vi "Contour Constructor.vi"(4 "Plot ID":i32, 6 "z matrix":sgl[][](array[numeric]), 8 "error in (no error)":errorcluster, 9 "y vector":sgl[][](array[numeric]), 10 "x vector":sgl[][](array[numeric]), 11 "3D Contour Datatype.lvclass in":refnum<class "3D Contour Datatype.lvclass">) -> (0 "error out":errorcluster, 3 "3D Contour Datatype.lvclass out":refnum<class "3D Contour Datatype.lvclass">)   [LabVIEW 2017, in "3D Contour Datatype.lvclass"]
uses:
  <vilib>/Math Plots/3D Math Plots/3D Contour/3D Contour Datatype/3D Contour Datatype.lvclass
  <vilib>/Math Plots/3D Math Plots/3D Contour/3D Contour Datatype/3D Contour Datatype.lvclass/3D Contour Datatype.ctl
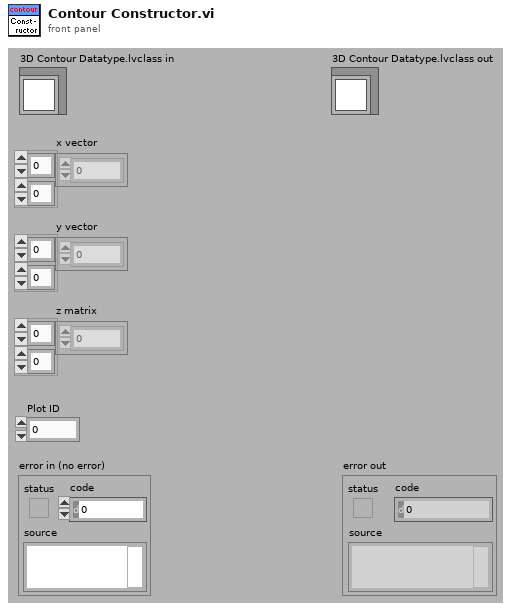
[diagram p1: front panel]
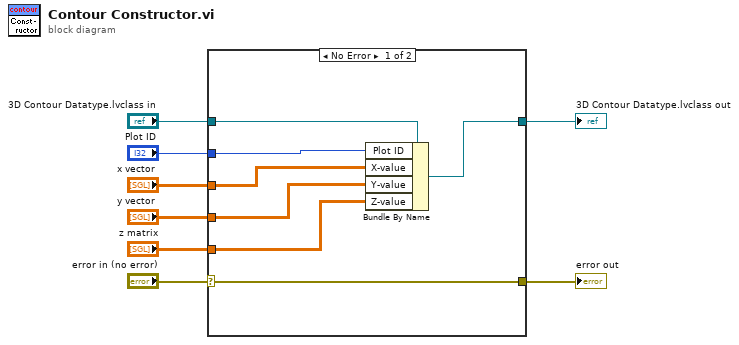
[diagram p0: block diagram]
diagram:
  n1 = case shown="No Error" "error in (no error)" {
    selector: "error in (no error)" -> [w10 w17]
    tunnel: "Plot ID" -> [w9 _]
    tunnel: [w10 w17] -> w7
    tunnel: "x vector" -> [w15 _]
    tunnel: "y vector" -> [w14 _]
    tunnel: "z matrix" -> [w13 _]
    tunnel: "3D Contour Datatype.lvclass in" -> [w12 w16]
    tunnel: [w11 w16] -> w1
    frame No Error {
      n2 = Bundle By Name(cluster=w12, "Plot ID"=w9, "X-value"=w15, "Y-value"=w14, "Z-value"=w13) -> (w11:refnum<class "3D Contour Datatype.lvclass">)
    }
    frame Error {
    }
  }
  "error out" <- w7
  "3D Contour Datatype.lvclass out" <- w1
